vi "new itc and dmm file 2.vi"() -> ()   [LabVIEW 2009]
panel:
  out "source out":string
  out "message":string
  out "error out":errorcluster
  out "error?":bool
  out "Sensor Resistance":dynamicdata(graph)
  out "Sensors Temperature":dynamicdata(graph)
  out "Resistance":dynamicdata(graph)
  out "Temperature":dynamicdata(graph)
  out "Measurement":bool caption="Taken"
  in  "stop":bool
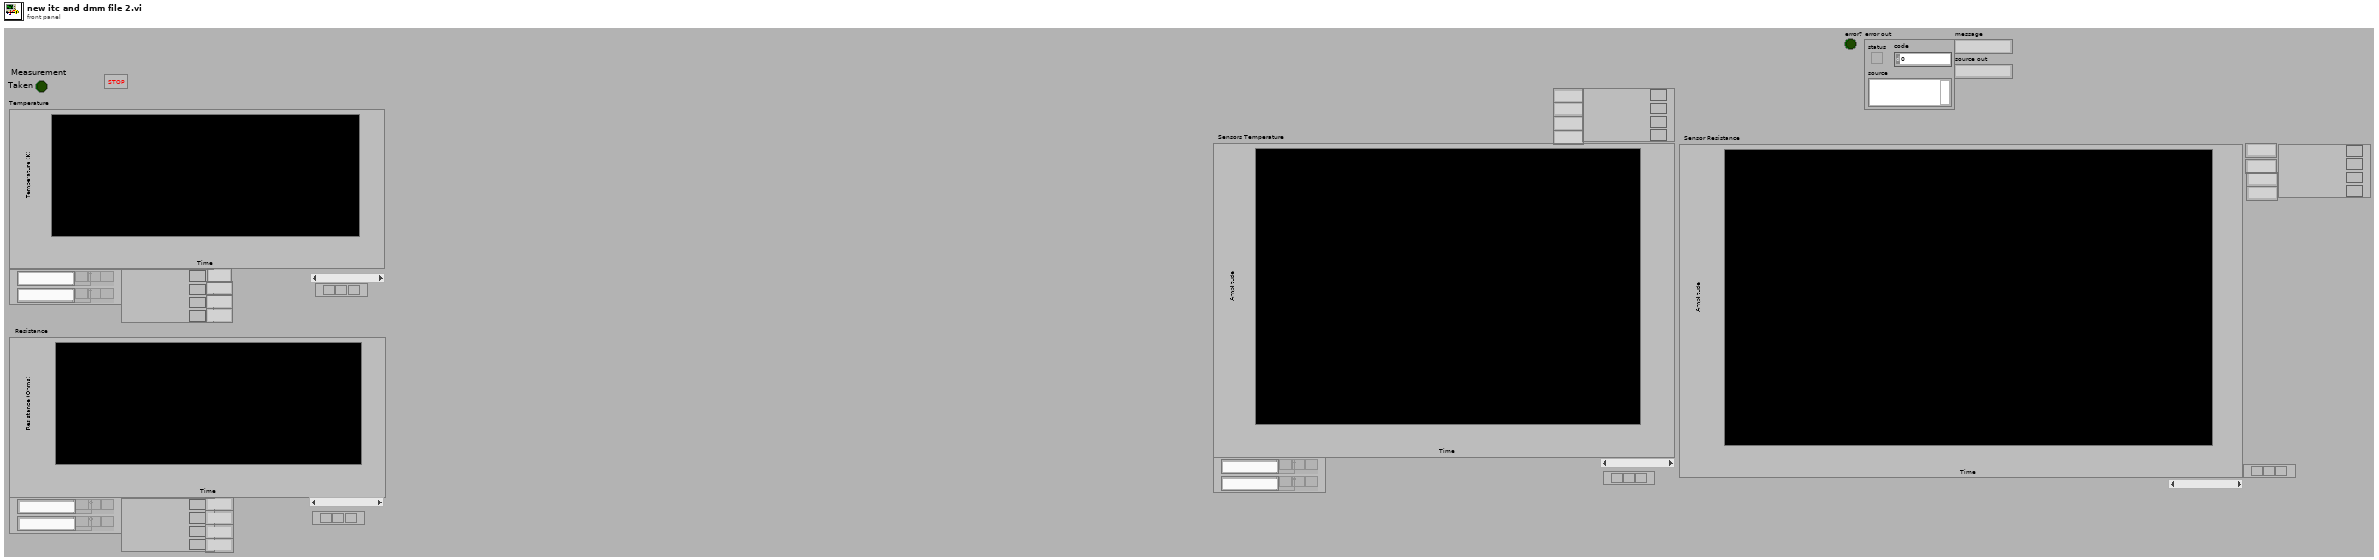
[diagram p1: front panel]
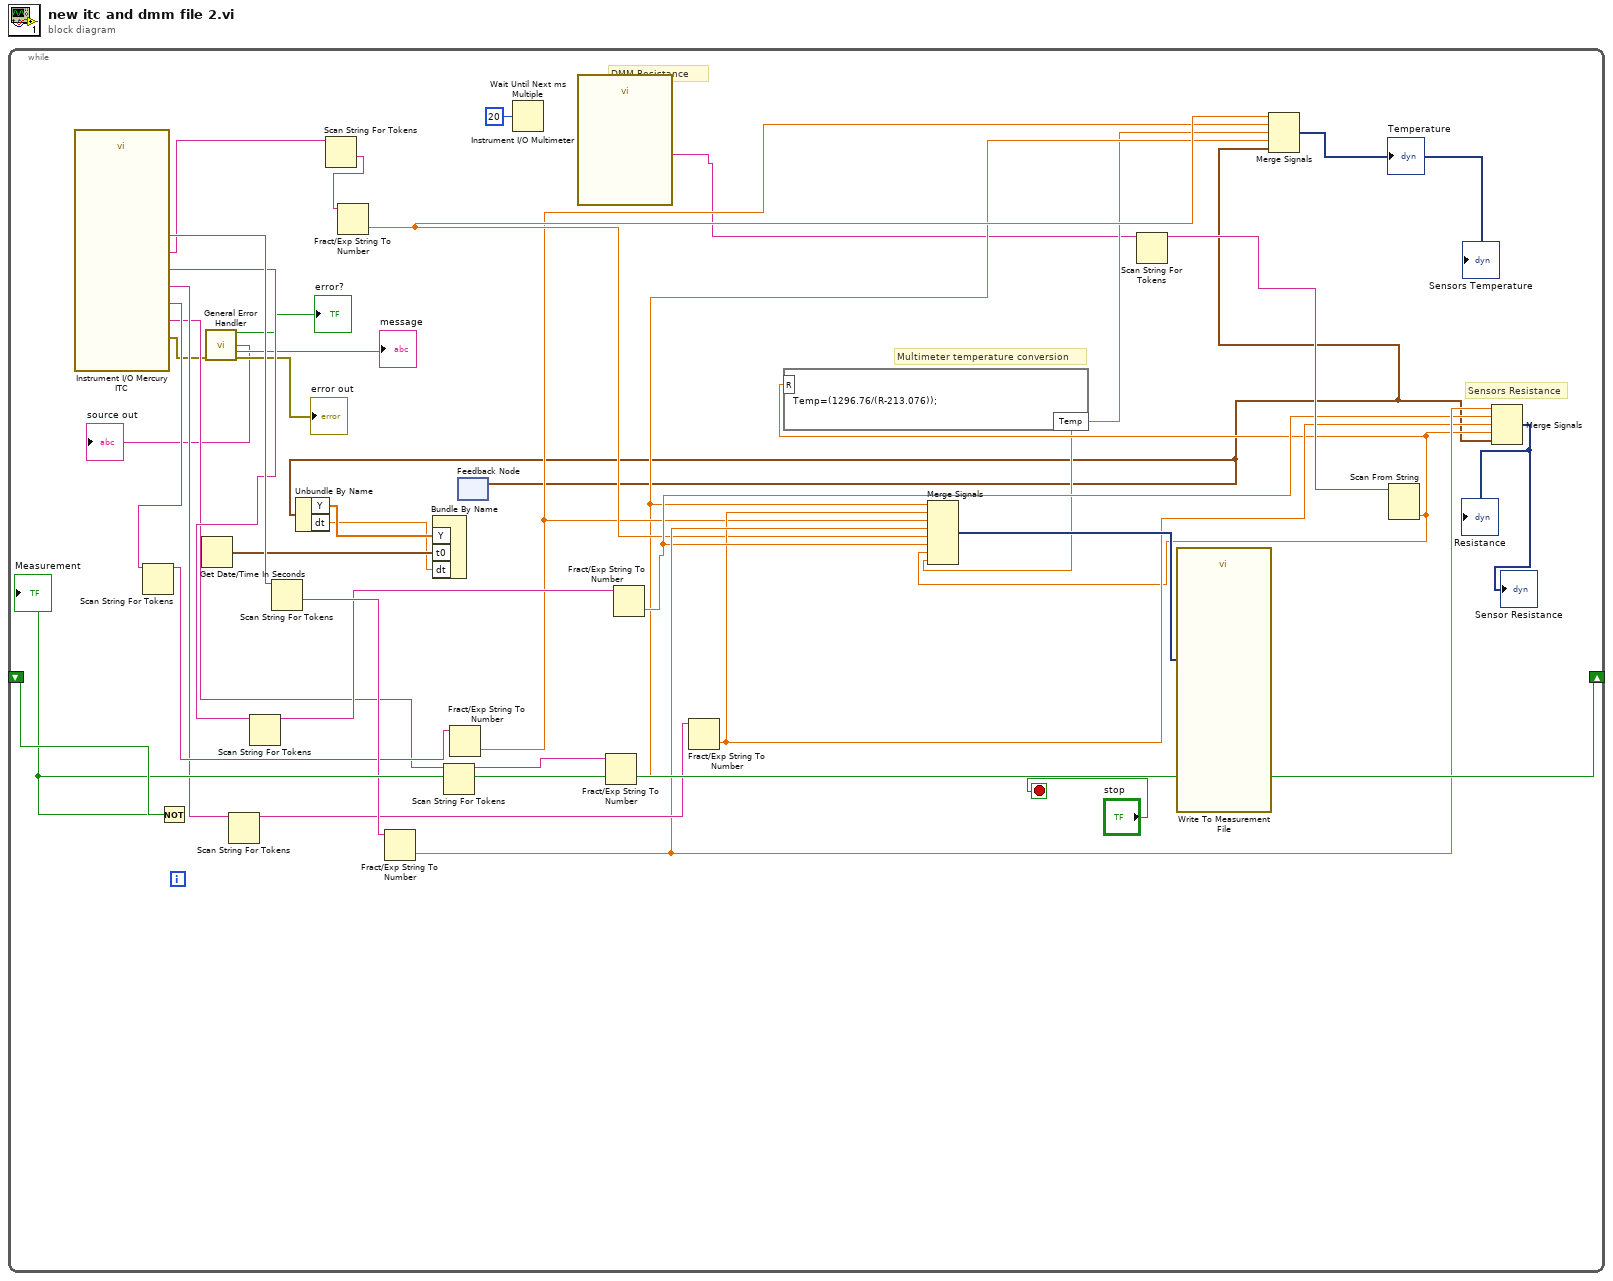
[diagram p0: block diagram]
diagram:
  n1 = while {
    shift-right: [w38] -> _
    shift-left: _ -> [w39]
    stop <- "stop" stop-if-true
    # "DMM Resistance"
    # "Sensors Resistance"
    # "Multimeter temperature conversion"
    n2 = call "Instrument I/O Mercury ITC"() -> ("CCS Resistance"=w28:string, "CCS Temperature"=w26:string, "Allen Bradley Temperature"=w30:string, "Allen Bradley Resistance"=w32:string, "Cernox Temp"=w1:string, "Cernox Resistance"=w37:string, "error out"=w8:errorcluster)  [unwired: 21 in]
    n3 = Scan String For Tokens(9:w30) -> (3:w29:string)  [unwired: 5 in, 3 out]
    n4 = Not(x=w39) -> (.not. x?=w38:bool)
    "Measurement" <- w38
    n5 = Get Date/Time In Seconds() -> (seconds since 1Jan1904=w33:timestamp)
    n6 = call <vilib>:"General Error Handler.vi"("error in (no error)"=w8) -> ("error?"=→"error?":bool, "source out"=→"source out":string, "message"=→"message":string, "error out"=→"error out":errorcluster)  [unwired: 10 in, 1 out]
    n7 = Scan String For Tokens(9:w28) -> (3:w27:string)  [unwired: 5 in, 3 out]
    n8 = Scan String For Tokens(9:w32) -> (3:w31:string)  [unwired: 5 in, 3 out]
    n9 = Scan String For Tokens(9:w37) -> (1:w36:string)  [unwired: 5 in, 3 out]
    n10 = Scan String For Tokens(9:w1) -> (1:w34:string)  [unwired: 5 in, 3 out]
    n11 = Fract/Exp String To Number(string=w34) -> (number=w18:dbl)  [unwired: 3 in, 1 out]
    n12 = Fract/Exp String To Number(string=w36) -> (number=w22:dbl)  [unwired: 3 in, 1 out]
    n13 = Scan String For Tokens(9:w26) -> (3:w25:string)  [unwired: 5 in, 3 out]
    n14 = Fract/Exp String To Number(string=w29) -> (number=w17:dbl)  [unwired: 3 in, 1 out]
    n15 = feedback #1() -> (w11:waveform(dbl))  [unwired: 1 in]
    n16 = Unbundle By Name(w11) -> ("Y"=w14:dbl[], "dt"=w13:dbl)
    n17 = Bundle By Name("Y"=w14, "t0"=w33, "dt"=w13) -> (w12:waveform(dbl))  [unwired: 1 in]
    n18 = Wait Until Next ms Multiple(millisecond multiple=u32 20) -> ()  [unwired: 1 out]
    n19 = call "Instrument I/O Multimeter"() -> ("Sample rate"=w2:string)  [unwired: 26 in, 1 out]
    n20 = Fract/Exp String To Number(string=w25) -> (number=w16:dbl)  [unwired: 3 in, 1 out]
    n21 = Fract/Exp String To Number(string=w31) -> (number=w21:dbl)  [unwired: 3 in, 1 out]
    n22 = Fract/Exp String To Number(string=w27) -> (number=w20:dbl)  [unwired: 3 in, 1 out]
    n23 = Scan String For Tokens(9:w2) -> (3:w23:string)  [unwired: 5 in, 3 out]
    n24 = Scan From String(input string=w23) -> (output 1=w19:dbl)  [unwired: 4 in, 3 out]
    n25 = formula code="Temp=(1296.76/(R-213.076));"("R"=w19) -> ("Temp"=w15:dbl)
    n26 = Merge Signals(w16, w20, w17, w22, w18, w21, w19, w15) -> (w35:dynamicdata)
    n27 = call "Write To Measurement File"("Signals"=w35) -> ()  [unwired: 16 in, 3 out]
    n28 = Merge Signals(w18, w17, w15, w16, w11) -> (→"Temperature" →"Sensors Temperature":dynamicdata)
    n29 = Merge Signals(w22, w21, w20, w19, w11) -> (→"Resistance" →"Sensor Resistance":dynamicdata)
  }
